vi "SetDisplayMode.vi"(8 "Error In":errorcluster, 11 "Keithley 6482 In":refnum<visa-resource-name>) -> (0 "Error Out":errorcluster, 3 "Keithley 6482 Out":refnum<visa-resource-name>)   [LabVIEW 2014, in "Keithley-6482-Visa.lvlib"]
uses:
  Keithley-6482-Visa.lvlib
  Controls/DisplayMode.ctl
panel:
  in  "Display Mode":T1=enum."DUAL"
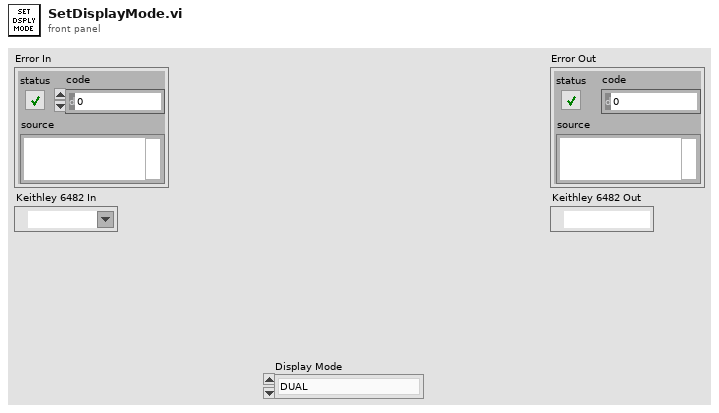
[diagram p1: front panel]
types:
  T1 = typedef "Keithley-6482-Visa.lvlib/DisplayMode.ctl" = enum16{"CALC3", "CALC4", "CALC5", "CALC6", "DUAL"}
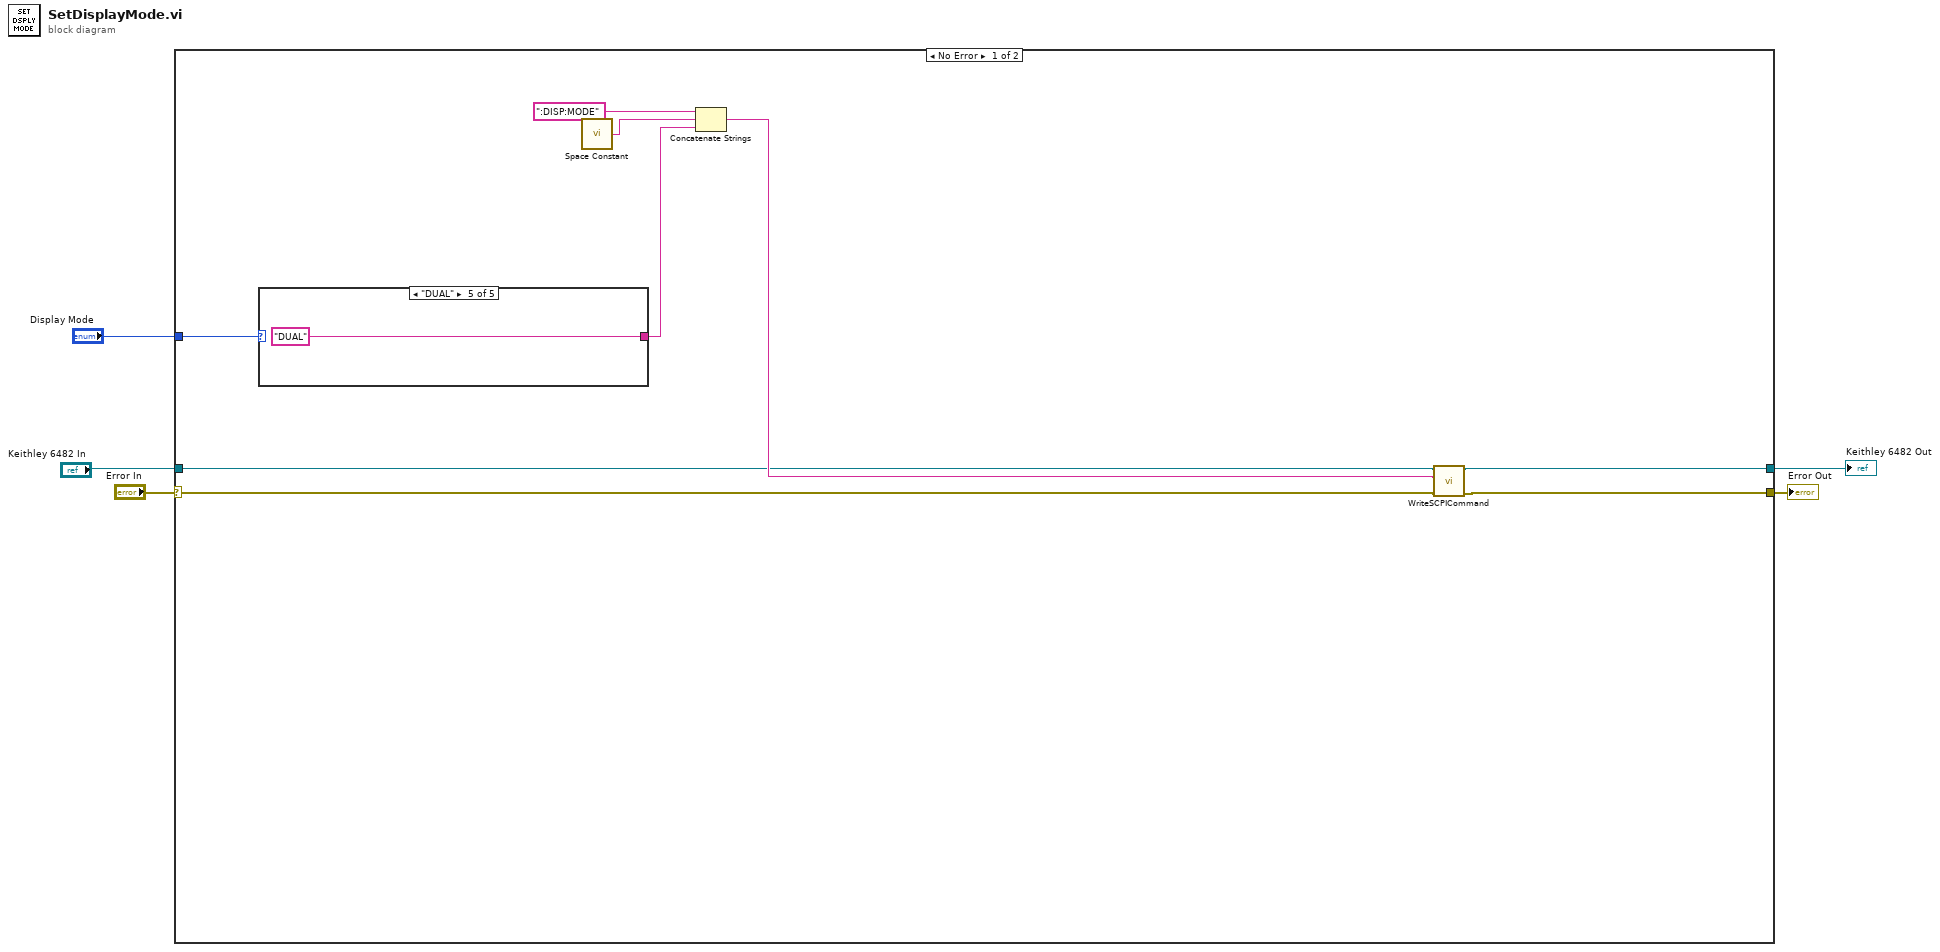
[diagram p0: block diagram]
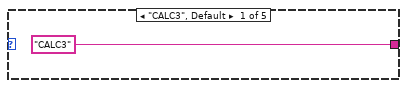
[diagram p2: hidden frame]
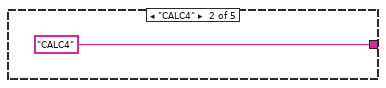
[diagram p3: hidden frame]
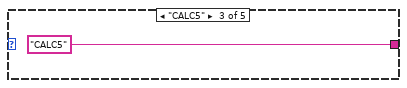
[diagram p4: hidden frame]
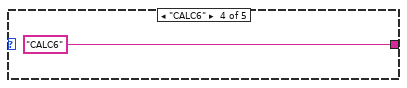
[diagram p5: hidden frame]
diagram:
  n1 = case shown="No Error" "Error In" {
    selector: "Error In" -> [w8 w20]
    tunnel: [w9 w20] -> w4
    tunnel: [w10 w21] -> w3
    tunnel: "Keithley 6482 In" -> [w6 w21]
    tunnel: "Display Mode" -> [w12 _]
    frame No Error {
      n2 = case shown="\"DUAL\"" w12 {
        tunnel: ["CALC3" "CALC4" "CALC5" "CALC6" "DUAL"] -> w11
        frame "CALC3", Default {
        }
        frame "CALC4" {
        }
        frame "CALC5" {
        }
        frame "CALC6" {
        }
        frame "DUAL" {
        }
      }
      n3 = call <vilib>:"Space Constant.vi"() -> ("String"=w13:string)
      n4 = Concatenate Strings(":DISP:MODE", w13, w11) -> (w7:string)
      n5 = call "WriteSCPICommand.vi"("Error In"=w8, "SCPI Command"=w7, "Keithley 6482 In"=w6) -> ("Error Out"=w9:errorcluster, "Keithley 6482 Out"=w10:refnum<visa-resource-name>)  [unwired: 7 in]
    }
    frame Error {
    }
  }
  "Error Out" <- w4
  "Keithley 6482 Out" <- w3
